vi "习题7.2.vi"() -> ()   [LabVIEW 2017]
panel:
  out "波形图":dbl[][](graph)
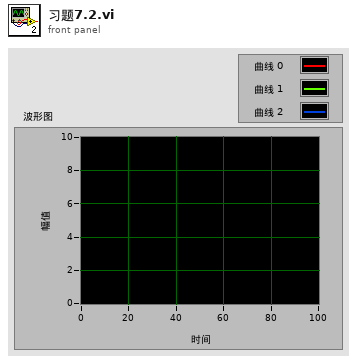
[diagram p1: front panel]
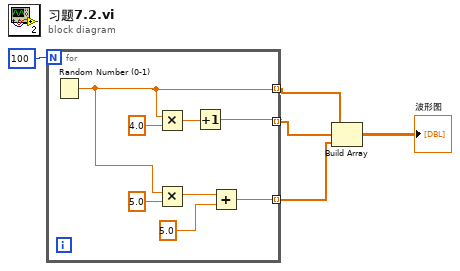
[diagram p0: block diagram]
diagram:
  n1 = for {
    N: 100 -> [_]
    tunnel: [w9] -> w4 mode=indexing
    tunnel: [w11] -> w3 mode=indexing
    tunnel: [w6] -> w2 mode=indexing
    n2 = Random Number (0-1)() -> (number: 0 to 1=w9:dbl)
    n3 = Multiply(x=w9, y=4.0) -> (x*y=w12:dbl)
    n4 = Multiply(x=w9, y=5.0) -> (x*y=w8:dbl)
    n5 = Increment(x=w12) -> (x+1=w11:dbl)
    n6 = Add(x=w8, y=5.0) -> (x+y=w6:dbl)
  }
  n7 = Build Array(w4, w3, w2) -> (→"波形图":dbl[][])
